vi "hasPacketIdentifier.vi"(11 "UNSUBSCRIBE in":refnum<class "UNSUBSCRIBE.lvclass">) -> (2 "As Packet Identifier":bool, 3 "UNSUBSCRIBE out":refnum<class "UNSUBSCRIBE.lvclass">)   [LabVIEW 2013, in "UNSUBSCRIBE.lvclass"]
uses:
  UNSUBSCRIBE.lvclass
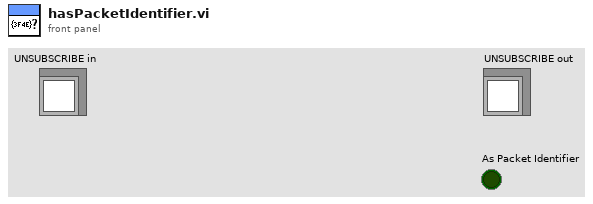
[diagram p1: front panel]
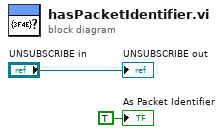
[diagram p0: block diagram]
diagram:
  "UNSUBSCRIBE out" <- "UNSUBSCRIBE in"
  "As Packet Identifier" <- TRUE ("As Packet Identifier")
